vi "Send.vi"(8 "error in (no error)":errorcluster, 10 "Send Notifier":refnum<notifier>) -> (0 "error out":errorcluster)   [LabVIEW 2022 SP3]
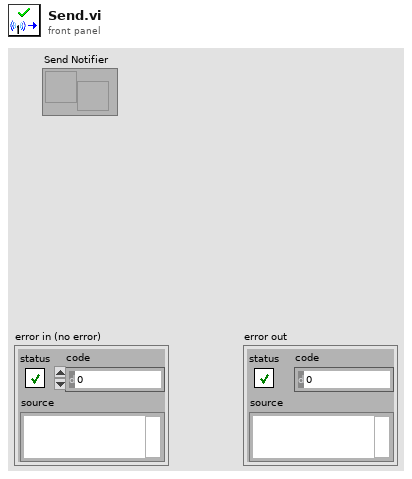
[diagram p1: front panel]
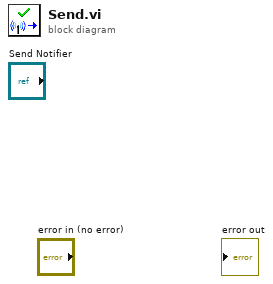
[diagram p0: block diagram]
diagram:
